vi "生成CODMn data (子VI).vi"() -> (3 "data":T1)   [LabVIEW 2016, in "斯坦道CODMn.lvlib"]
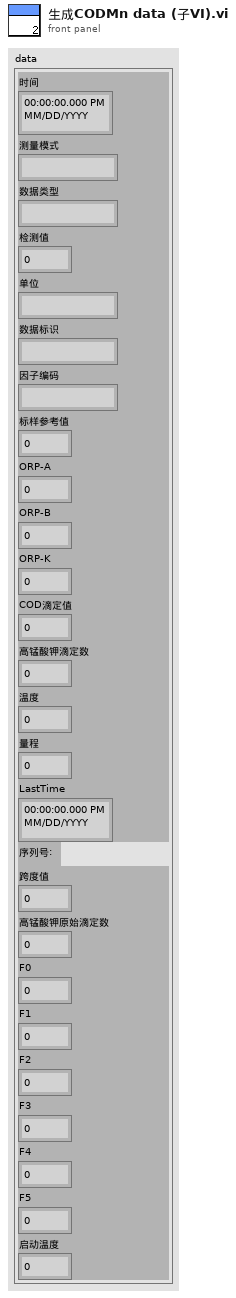
[diagram p1: front panel]
types:
  T1 = cluster{"时间":timestamp, "测量模式":string, "数据类型":string, "检测值":sgl, "单位":string, "数据标识":string, "因子编码":string, "标样参考值":sgl, "ORP-A":sgl, "ORP-B":sgl, "ORP-K":sgl, "COD滴定值":sgl, "高锰酸钾滴定数":sgl, "温度":sgl, "量程":sgl, "LastTime":timestamp, "序列号:":string, "跨度值":sgl, "高锰酸钾原始滴定数":sgl, "F0":sgl, "F1":sgl, "F2":sgl, "F3":sgl, "F4":sgl, "F5":sgl, "启动温度":sgl}
  T2 = cluster{"数组 2[0]":sgl, "数组 2[1]":sgl, "数组 2[2]":sgl, "数组 2[3]":sgl, "数组 2[4]":sgl, "数组 2[5]":sgl, "数组 2[6]":sgl, "数组 2[7]":sgl, "数组 2[8]":sgl, "数组 2[9]":sgl, "数组 2[10]":sgl, "数组 2[11]":sgl, "数组 2[12]":sgl, "数组 2[13]":sgl, "数组 2[14]":sgl, "数组 2[15]":sgl, "数组 2[16]":sgl, "数组 2[17]":sgl, "数组 2[18]":sgl, "数组 2[19]":sgl, "数组 2[20]":sgl, "数组 2[21]":sgl, "数组 2[22]":sgl, "数组 2[23]":sgl, "数组 2[24]":sgl, "数组 2[25]":sgl, "数组 2[26]":sgl, "数组 2[27]":sgl, "数组 2[28]":sgl, "数组 2[29]":sgl, "数组 2[30]":sgl, "数组 2[31]":sgl, "数组 2[32]":sgl, "数组 2[33]":sgl, "数组 2[34]":sgl, "数组 2[35]":sgl, "数组 2[36]":sgl, "数组 2[37]":sgl, "数组 2[38]":sgl, "数组 2[39]":sgl, "数组 2[40]":sgl, "数组 2[41]":sgl}
  T3 = cluster{"运行模式":enum16{"维护模式", "常规模式", "应急模式", "质控模式"}, "质控频次":enum16{"关闭", "每天", "星期一", "星期二", "星期三", "星期四", "星期五", "星期六", "星期日"}, "空白核查时间":u16, "跨度核查时间":u16, "测量间隔":u16}
  T4 = cluster{"测量量程":dbl, "测量精度":dbl, "测量间隔":dbl, "消解温度":dbl, "消解时长":dbl, "空白校准时间":timestamp, "曲线截距":dbl, "曲线斜率":dbl, "测量检出限":dbl, "测量信号值":dbl, "线性相关系数":dbl, "二次多项式系数":dbl, "标样校准时间":timestamp, "稀释倍数":dbl, "三项式系数":dbl, "空白标定系数":dbl, "量程系数":dbl, "F0/ORPA":dbl, "F1/ORPB":dbl, "F2/ORPK":dbl, "F3":dbl, "F4":dbl, "F5":dbl, "F6":dbl, "F7":dbl, "X0/滴定数":dbl, "量程":dbl}
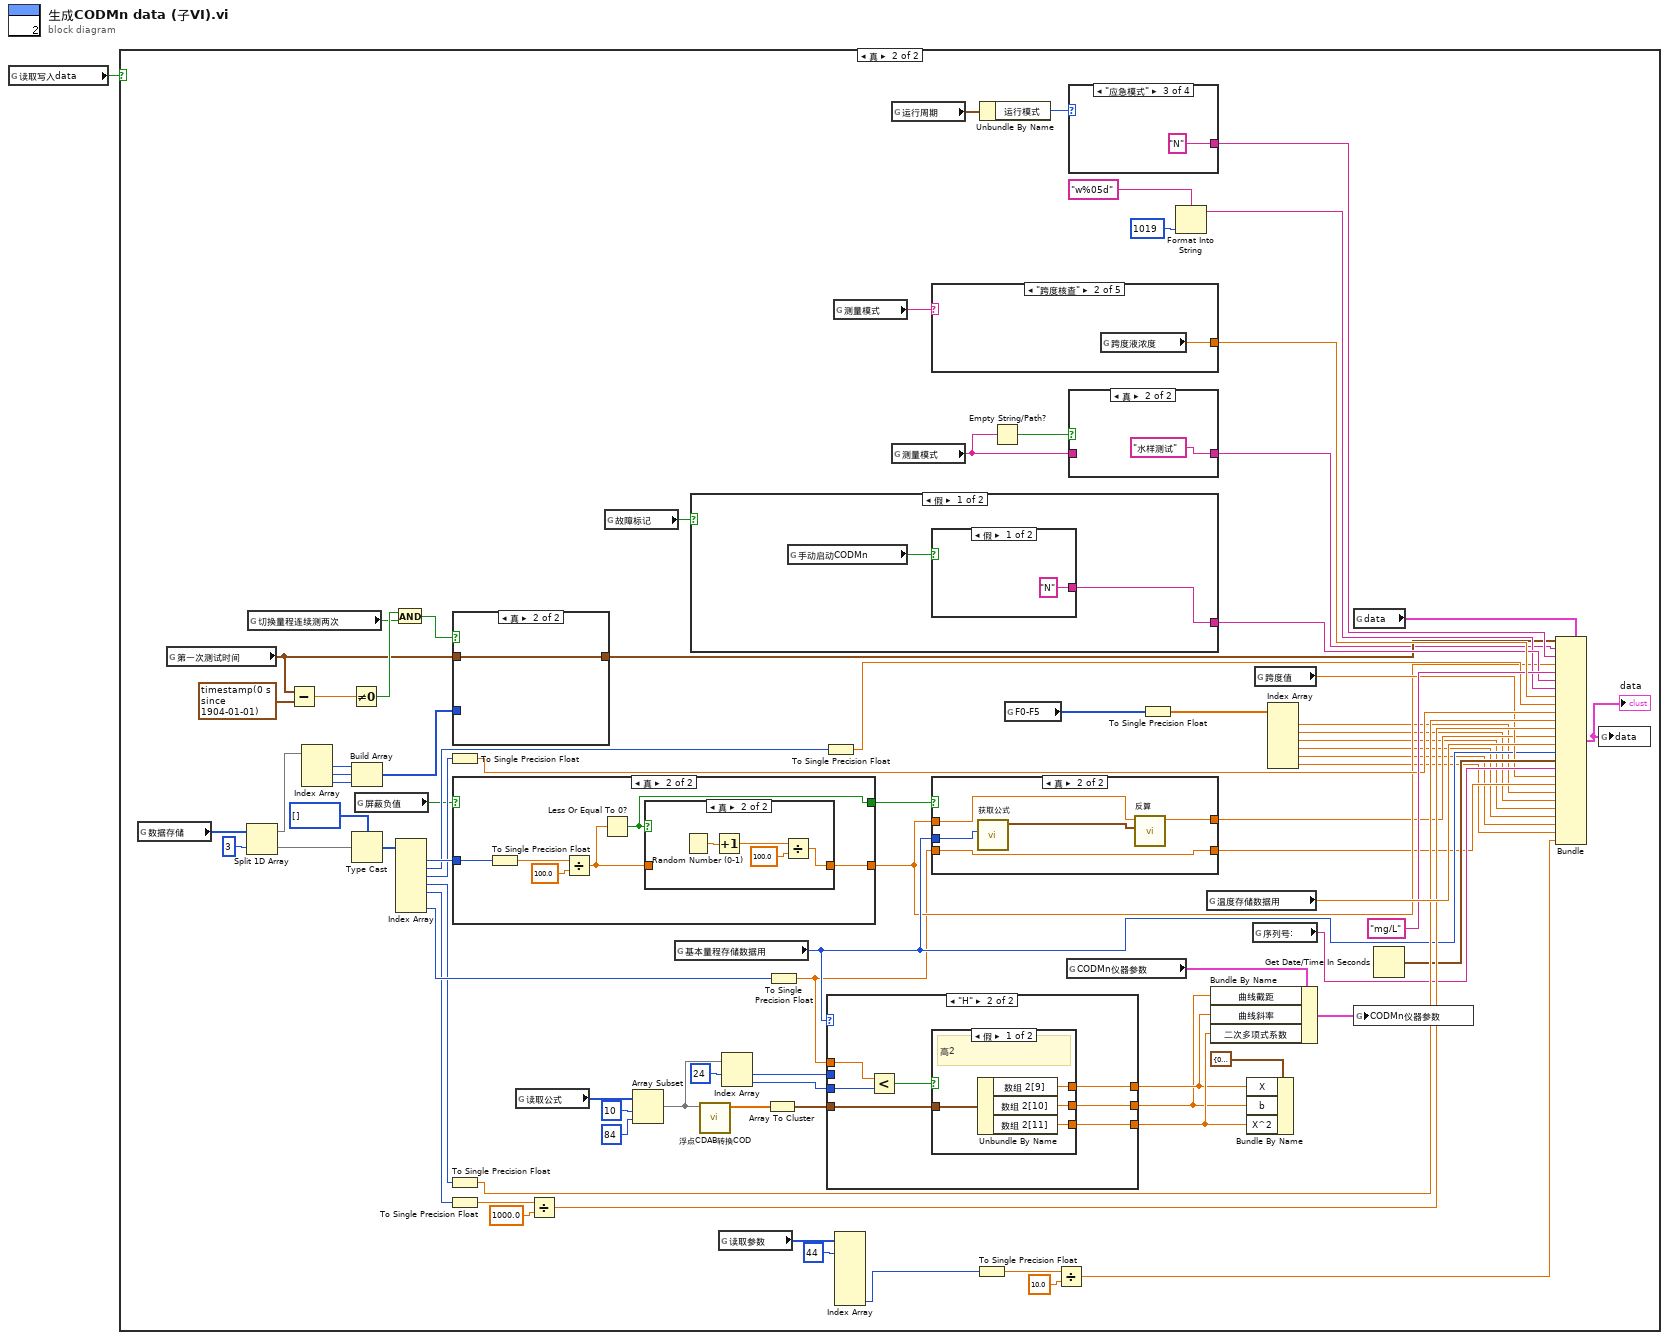
[diagram p0: block diagram]
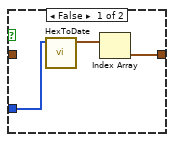
[diagram p3: hidden frame]
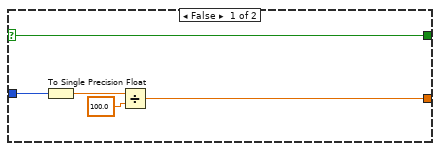
[diagram p5: hidden frame]
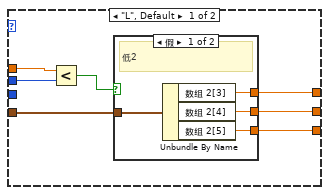
[diagram p8: hidden frame]
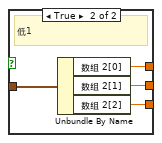
[diagram p9: hidden frame]
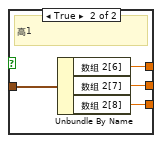
[diagram p10: hidden frame]
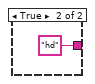
[diagram p11: hidden frame]
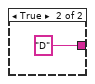
[diagram p12: hidden frame]
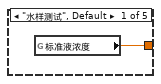
[diagram p13: hidden frame]
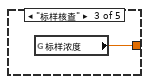
[diagram p14: hidden frame]
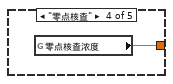
[diagram p15: hidden frame]
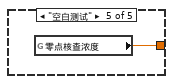
[diagram p16: hidden frame]
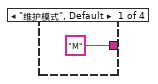
[diagram p17: hidden frame]
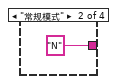
[diagram p18: hidden frame]
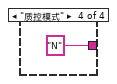
[diagram p19: hidden frame]
diagram:
  n1 = global read "COD内部交互全局.vi" "读取写入data"() -> (w1:bool)
  n2 = case shown="真" w1 {
    frame False {
    }
    frame True {
      n3 = global read "COD内部交互全局.vi" "数据存储"() -> (w57:u16[])
      n4 = global read "COD内部交互全局.vi" "第一次测试时间"() -> (w16:timestamp)
      n5 = Split 1D Array(array=w57, index=3 ("索引")) -> (first subarray=w61:u16[], second subarray=w56:u16[])
      n6 = global read "COD内部交互全局.vi" "切换量程连续测两次"() -> (w18:bool)
      n7 = Subtract(x=w16, y=timestamp(0 s since 1904-01-01) ("第一次测试时间")) -> (x-y=w20:dbl)
      n8 = Index Array(array=w61) -> (element #1=w62:u16, element #2=w63:u16, element #3=w64:u16)  [unwired: 3 in]
      n9 = Not Equal To 0?(x=w20) -> (x != 0?=w19:bool)
      n10 = Build Array(w62, w63, w64) -> (w65:u16[])
      n11 = Type Cast(type=i16[] [], x=w56) -> (*(type *) &x=w55:i16[])
      n12 = global read "CODMn断电保存全局变量.vi" "屏蔽负值"() -> (w27:bool)
      n13 = And(x=w19, y=w18) -> (x .and. y?=w17:bool)
      n14 = Index Array(array=w55) -> (element #1=w82:i16, element #2=w66:i16, element #3=w67:i16, element #4=w68:i16, element #5=w69:i16, element #7=w84:i16)  [unwired: 7 in, 1 out]
      n15 = To Single Precision Float(number=w67) -> (single precision float=w76:sgl)
      n16 = To Single Precision Float(number=w68) -> (single precision float=w75:sgl)
      n17 = To Single Precision Float(number=w69) -> (single precision float=w72:sgl)
      n18 = case shown="真" w17 {
        tunnel: w65 -> [w89 _]
        tunnel: [w87 w90] -> w54
        tunnel: w16 -> [_ w90]
        frame False {
          n19 = call "HexToDate.vi"("数组"=w89) -> ("DATE"=w88:timestamp[])  [unwired: 10 in]
          n20 = Index Array(array=w88) -> (element=w87:timestamp)  [unwired: 1 in]
        }
        frame True {
        }
      }
      n21 = case shown="真" w27 {
        selector: w27 -> [w93 _]
        tunnel: w82 -> [w95 w100]
        tunnel: [w94 w103] -> w31
        tunnel: [w93 w99] -> w28
        frame False {
          n22 = To Single Precision Float(number=w95) -> (single precision float=w97:sgl)
          n23 = Divide(x=w97, y=sgl 100.0) -> (x/y=w94:sgl)
        }
        frame True {
          n24 = To Single Precision Float(number=w100) -> (single precision float=w101:sgl)
          n25 = Divide(x=w101, y=sgl 100.0) -> (x/y=w98:sgl)
          n26 = Less Or Equal To 0?(x=w98) -> (x <= 0?=w99:bool)
          n27 = case shown="真" w99 {
            tunnel: [w104 w108] -> w103
            tunnel: w98 -> [w104 _]
            frame False {
            }
            frame True {
              n28 = Random Number (0-1)() -> (number: 0 to 1=w107:dbl)
              n29 = Increment(x=w107) -> (x+1=w105:dbl)
              n30 = Divide(x=w105, y=sgl 100.0) -> (x/y=w108:dbl)
            }
          }
        }
      }
      n31 = global read "COD内部交互全局.vi" "读取公式"() -> (w43:u16[])
      n32 = Divide(x=w72, y=sgl 1000.0) -> (x/y=w74:sgl)
      n33 = global read "COD内部交互全局.vi" "故障标记"() -> (w86:bool)
      n34 = Array Subset(array=w43, index=10 ("索引"), length=84 ("长度")) -> (w39:u16[])
      n35 = global read "COD内部交互全局.vi" "基本量程存储数据用"() -> (w32:enum16{"L", "H", "AUTO"})
      n36 = case shown="假" w86 {
        tunnel: [w146 "D" ("数据标识")] -> w79
        frame False {
          n37 = global read "CODMN外部API.vi" "手动启动CODMn"() -> (w145:bool)
          n38 = case shown="假" w145 {
            tunnel: ["N" ("数据标识") "hd" ("数据标识")] -> w146
            frame False {
            }
            frame True {
            }
          }
        }
        frame True {
        }
      }
      n39 = call "浮点CDAB转换COD.vi"("数组"=w39) -> ("数组 2"=w42:sgl[])  [unwired: 10 in]
      n40 = global read "COD内部交互全局.vi" "读取参数"() -> (w7:u16[])
      n41 = Index Array(array=w39, index #1=24 ("索引")) -> (element #1=w45:u16, element #2=w46:u16)  [unwired: 1 in]
      n42 = Array To Cluster(array=w42) -> (cluster=w44:T2)
      n43 = To Single Precision Float(number=w84) -> (single precision float=w29:sgl)
      n44 = To Single Precision Float(number=w66) -> (single precision float=w77:sgl)
      n45 = case shown="\"H\"" w32 {
        tunnel: w44 -> [w118 w135]
        tunnel: w45 -> [w120 _]
        tunnel: w46 -> [_ w133]
        tunnel: w29 -> [w121 w134]
        tunnel: [w117 w132] -> w34
        tunnel: [w116 w131] -> w33
        tunnel: [w115 w130] -> w35
        frame "L", Default {
          n46 = Less?(x=w121, y=w120) -> (x < y?=w119:bool)
          n47 = case shown="假" w119 {
            tunnel: w118 -> [w125 w129]
            tunnel: [w124 w128] -> w117
            tunnel: [w123 w127] -> w116
            tunnel: [w122 w126] -> w115
            frame False {
              # "低2"
              n48 = Unbundle By Name(w125) -> ("数组 2[3]"=w124:sgl, "数组 2[4]"=w123:sgl, "数组 2[5]"=w122:sgl)
            }
            frame True {
              # "低1"
              n49 = Unbundle By Name(w129) -> ("数组 2[0]"=w128:sgl, "数组 2[1]"=w127:sgl, "数组 2[2]"=w126:sgl)
            }
          }
        }
        frame "H" {
          n50 = Less?(x=w134, y=w133) -> (x < y?=w136:bool)
          n51 = case shown="假" w136 {
            tunnel: w135 -> [w140 w144]
            tunnel: [w139 w143] -> w132
            tunnel: [w138 w142] -> w131
            tunnel: [w137 w141] -> w130
            frame False {
              # "高2"
              n52 = Unbundle By Name(w140) -> ("数组 2[9]"=w139:sgl, "数组 2[10]"=w138:sgl, "数组 2[11]"=w137:sgl)
            }
            frame True {
              # "高1"
              n53 = Unbundle By Name(w144) -> ("数组 2[6]"=w143:sgl, "数组 2[7]"=w142:sgl, "数组 2[8]"=w141:sgl)
            }
          }
        }
      }
      n54 = global read "CODMn断电保存全局变量.vi" "测量模式"() -> (w22:string)
      n55 = Index Array(array=w7, index #1=44 ("索引")) -> (element #7=w3:u16)  [unwired: 6 in, 6 out]
      n56 = global read "CODMn断电保存全局变量.vi" "运行周期"() -> (w51:T3)
      n57 = global read "CODMn断电保存全局变量.vi" "测量模式"() -> (w23:string)
      n58 = case shown="\"跨度核查\"" w22 {
        tunnel: [w150 w151 w152 w153 w154] -> w83
        frame "水样测试", Default {
          n59 = global read "COD浓度全局变量.vi" "标准液浓度"() -> (w150:dbl)
        }
        frame "跨度核查" {
          n60 = global read "CODMn断电保存全局变量.vi" "跨度液浓度"() -> (w151:dbl)
        }
        frame "标样核查" {
          n61 = global read "CODMn断电保存全局变量.vi" "标样浓度"() -> (w152:dbl)
        }
        frame "零点核查" {
          n62 = global read "CODMn断电保存全局变量.vi" "零点核查浓度"() -> (w153:dbl)
        }
        frame "空白测试" {
          n63 = global read "CODMn断电保存全局变量.vi" "零点核查浓度"() -> (w154:dbl)
        }
      }
      n64 = case shown="真" w28 {
        tunnel: w32 -> [_ w113]
        tunnel: w31 -> [_ w112]
        tunnel: [w109 w111] -> w30
        tunnel: w29 -> [w109 w110]
        tunnel: [w109 w110] -> w26
        frame False {
        }
        frame True {
          n65 = call "获取公式.vi"("量程选择"=w113) -> ("方程系数"=w114:cluster{"X^2":dbl, "K":dbl, "b":dbl})  [unwired: 9 in, 1 out]
          n66 = call "反算.vi"("公式"=w114, "监测值"=w112) -> ("信号值"=w111:dbl)  [unwired: 8 in, 1 out]
        }
      }
      n67 = To Single Precision Float(number=w3) -> (single precision float=w4:sgl)
      n68 = Unbundle By Name(w51) -> ("运行模式"=w50:enum16{"维护模式", "常规模式", "应急模式", "质控模式"})
      n69 = Empty String/Path?(string/path=w23) -> (empty?=w25:bool)
      n70 = global read "COD内部交互全局.vi" "F0-F5"() -> (w15:u16[])
      n71 = Divide(x=w4, y=sgl 10.0) -> (x/y=w2:sgl)
      n72 = global read "CODMn断电保存全局变量.vi" "CODMn仪器参数"() -> (w37:T4)
      n73 = case shown="\"应急模式\"" w50 {
        tunnel: ["M" ("单位") "N" ("单位") "N" ("单位") "N" ("单位")] -> w81
        frame "维护模式", Default {
        }
        frame "常规模式" {
        }
        frame "应急模式" {
        }
        frame "质控模式" {
        }
      }
      n74 = case shown="真" w25 {
        tunnel: [w91 "水样测试" ("测量模式")] -> w24
        tunnel: w23 -> [w91 _]
        frame False {
        }
        frame True {
        }
      }
      n75 = To Single Precision Float(number=w15) -> (single precision float=w14:sgl[])
      n76 = Format Into String(format string="w%05d" ("格式字符串"), u32 1019 ("因子编码")) -> (resulting string=w78:string)  [unwired: 2 in, 1 out]
      n77 = global read "COD内部交互全局.vi" "温度存储数据用"() -> (w85:dbl)
      n78 = Bundle By Name(cluster=w37, "曲线截距"=w33, "曲线斜率"=w34, "二次多项式系数"=w35) -> (w36:T4)
      n79 = Bundle By Name(cluster=cluster{"X":dbl, "b":dbl, "X^2":dbl} {"X"=0.0, "b"=0.0, "X^2"=0.0} ("方程系数"), "X"=w34, "b"=w33, "X^2"=w35) -> ()  [unwired: 1 out]
      n80 = global read "COD内部交互全局.vi" "序列号:"() -> (w53:string)
      n81 = global read "CODMn断电保存全局变量.vi" "跨度值"() -> (w48:dbl)
      n82 = Index Array(array=w14) -> (element #1=w13:sgl, element #2=w12:sgl, element #3=w11:sgl, element #4=w10:sgl, element #5=w9:sgl, element #6=w8:sgl)  [unwired: 6 in]
      n83 = global read "COD内部交互全局.vi" "data"() -> (w49:T1)
      n84 = global write "CODMn断电保存全局变量.vi" "CODMn仪器参数"(w36) -> ()
      n85 = Get Date/Time In Seconds() -> (seconds since 1Jan1904=w59:timestamp)
      n86 = Bundle(cluster=w49, "时间"=w54, "测量模式"=w24, "数据类型"=w81, "检测值"=w31, "单位"="mg/L", "数据标识"=w79, "因子编码"=w78, "标样参考值"=w83, "ORP-A"=w77, "ORP-B"=w76, "ORP-K"=w75, "COD滴定值"=w74, "高锰酸钾滴定数"=w30, "温度"=w85, "量程"=w32, "LastTime"=w59, "序列号:"=w53, "跨度值"=w48, "高锰酸钾原始滴定数"=w26, "F0"=w13, "F1"=w12, "F2"=w11, "F3"=w10, "F4"=w9, "F5"=w8, "启动温度"=w2) -> (w52:T1)
      "data" <- w52
      n87 = global write "COD内部交互全局.vi" "data"(w52) -> ()
    }
  }
